vi "poly_is_poly_vi_path.vi"(2 "vi path":path) -> (7 "is poly vi?":bool)   [LabVIEW 2015]
uses:
  <vilib>/Utility/Data Type/Type Definitions/Data Type.ctl
  <vilib>/Utility/Data Type/NI_Data Type.lvlib
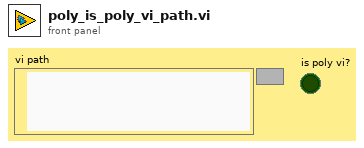
[diagram p1: front panel]
types:
  T1 = typedef "NI_Data Type.lvlib/Data Type.ctl" = enum8{"Invalid Type", "Void", "I8", "I16", "I32", "I64", "U8", "U16", "U32", "U64", "Single Float", "Double Float", "Extended Float", "Single Complex", "Double Complex", "Extended Complex", "Enum U8", "Enum U16", "Enum U32", "Enum U64", "Single Float With Unit", "Double Float With Unit", "Extended Float With Unit", "Single Complex with Unit", "Double Complex with Unit", "Extended Complex with Unit", "Boolean", "String", "Path", "Picture", "Tag", "Array", "Cluster", "Variant", "LV Variant", "Waveform", "Timestamp", "Digital Waveform", "Digital Data", "ExpressData", "Refnum", "External Data", "VI", "Poly VI", "LabVIEW Class Instance", "Fixed Point"}
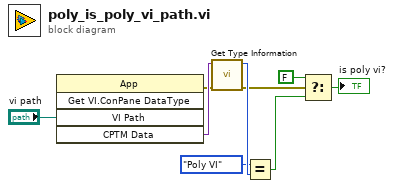
[diagram p0: block diagram]
diagram:
  n1 = invoke class="App" method="Get VI.ConPane DataType"("VI Path"="vi path") -> (error out=w7:errorcluster, "CPTM Data"=w8:variant)  [unwired: 4 in, 3 out]
  n2 = call <vilib>:"Get Type Information.vi"("error in (no error)"=w7, "Variant"=w8) -> ("error out"=w4:errorcluster, "Type"=w6:T1)  [unwired: 5 in, 3 out]
  n3 = Equal?(x=Data_Type."Poly VI" ("Type"), y=w6) -> (x = y?=w3:bool)
  n4 = Select(t=FALSE, s=w4, f=w3) -> (s? t:f=→"is poly vi?":bool)
